vi "_OBSOLETE_PathPlanner_Trajectory_JoinSplines.vi"(9 "Step":dbl, 10 "Max Velocity":dbl, 11 "PathPoints":T5[](array[typedef]) {"HolonomicRotation"."SIN" format="%13.4f"; "HolonomicRotation"."COS" format="%13.4f"; "HolonomicRotation"."VALUE" format="%13.4f"; "NextControl"."Y" format="%14.3f"; "NextControl"."X" format="%14.3f"; "PrevControl"."Y" format="%14.3f"; "PrevControl"."X" format="%14.3f"; "AnchorPoint"."Y" format="%14.3f"; "AnchorPoint"."X" format="%14.3f"}) -> (3 "outPathPlannerStates":T1[](array[typedef]) {"TargetHolonomicRotation"."SIN" format="%13.4f"; "TargetHolonomicRotation"."COS" format="%13.4f"; "TargetHolonomicRotation"."VALUE" format="%13.4f"; "Heading"."SIN" format="%13.4f"; "Heading"."COS" format="%13.4f"; "Heading"."VALUE" format="%13.4f"; "PositionMeters"."Y" format="%14.3f"; "PositionMeters"."X" format="%14.3f"})   [LabVIEW 2019]
uses:
  <vilib>/Rock Robotics/WPI/ThirdParty/JAS_Junk/TrajLib/TypeDef/ROTATION2D.ctl
  <vilib>/Rock Robotics/WPI/ThirdParty/JAS_Junk/TrajLib/Trajectory_Library.lvlib
  <vilib>/Rock Robotics/WPI/ThirdParty/JAS_Junk/TrajLib/TypeDef/TRANSLATION2D.ctl
  TypeDef/PathPlannerTrajectoryState.ctl
  PathPlanner24.lvlib
  TypeDef/PathPlannerPathConstraints.ctl
  TypeDef/PathPlannerWaypoint.ctl
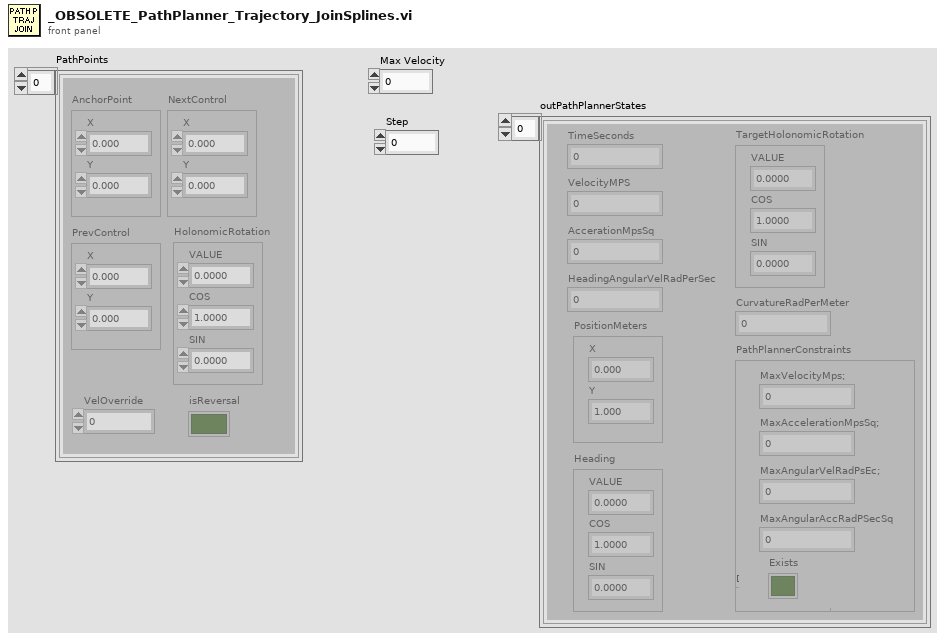
[diagram p1: front panel]
types:
  T1 = typedef "PathPlanner24.lvlib/PathPlannerTrajectoryState.ctl" = cluster{"TimeSeconds":dbl, "VelocityMPS":dbl, "AccerationMpsSq":dbl, "HeadingAngularVelRadPerSec":dbl, "PositionMeters":T2, "Heading":T3, "TargetHolonomicRotation":T3, "CurvatureRadPerMeter":dbl, "DeltaPos":dbl, "PathPlannerConstraints":T4}
  T2 = typedef "Trajectory_Library.lvlib/TRANSLATION2D.ctl" = cluster{"X":dbl, "Y":dbl}
  T3 = typedef "Trajectory_Library.lvlib/ROTATION2D.ctl" = cluster{"VALUE":dbl, "COS":dbl, "SIN":dbl}
  T4 = typedef "PathPlanner24.lvlib/PathPlannerPathConstraints.ctl" = cluster{"MaxVelocityMps;":dbl, "MaxAccelerationMpsSq;":dbl, "MaxAngularVelRadPsEc;":dbl, "MaxAngularAccRadPSecSq":dbl, "Exists":bool}
  T5 = typedef "PathPlanner24.lvlib/PathPlannerWaypoint.ctl" = cluster{"AnchorPoint":T2, "PrevControl":T2, "NextControl":T2, "HolonomicRotation":T3, "VelOverride":dbl, "isReversal":bool}
  T6 = typedef "Trajectory_Library.lvlib/POSE2D.ctl" = cluster{"TRANSLATION":T2, "ROTATION":T3}
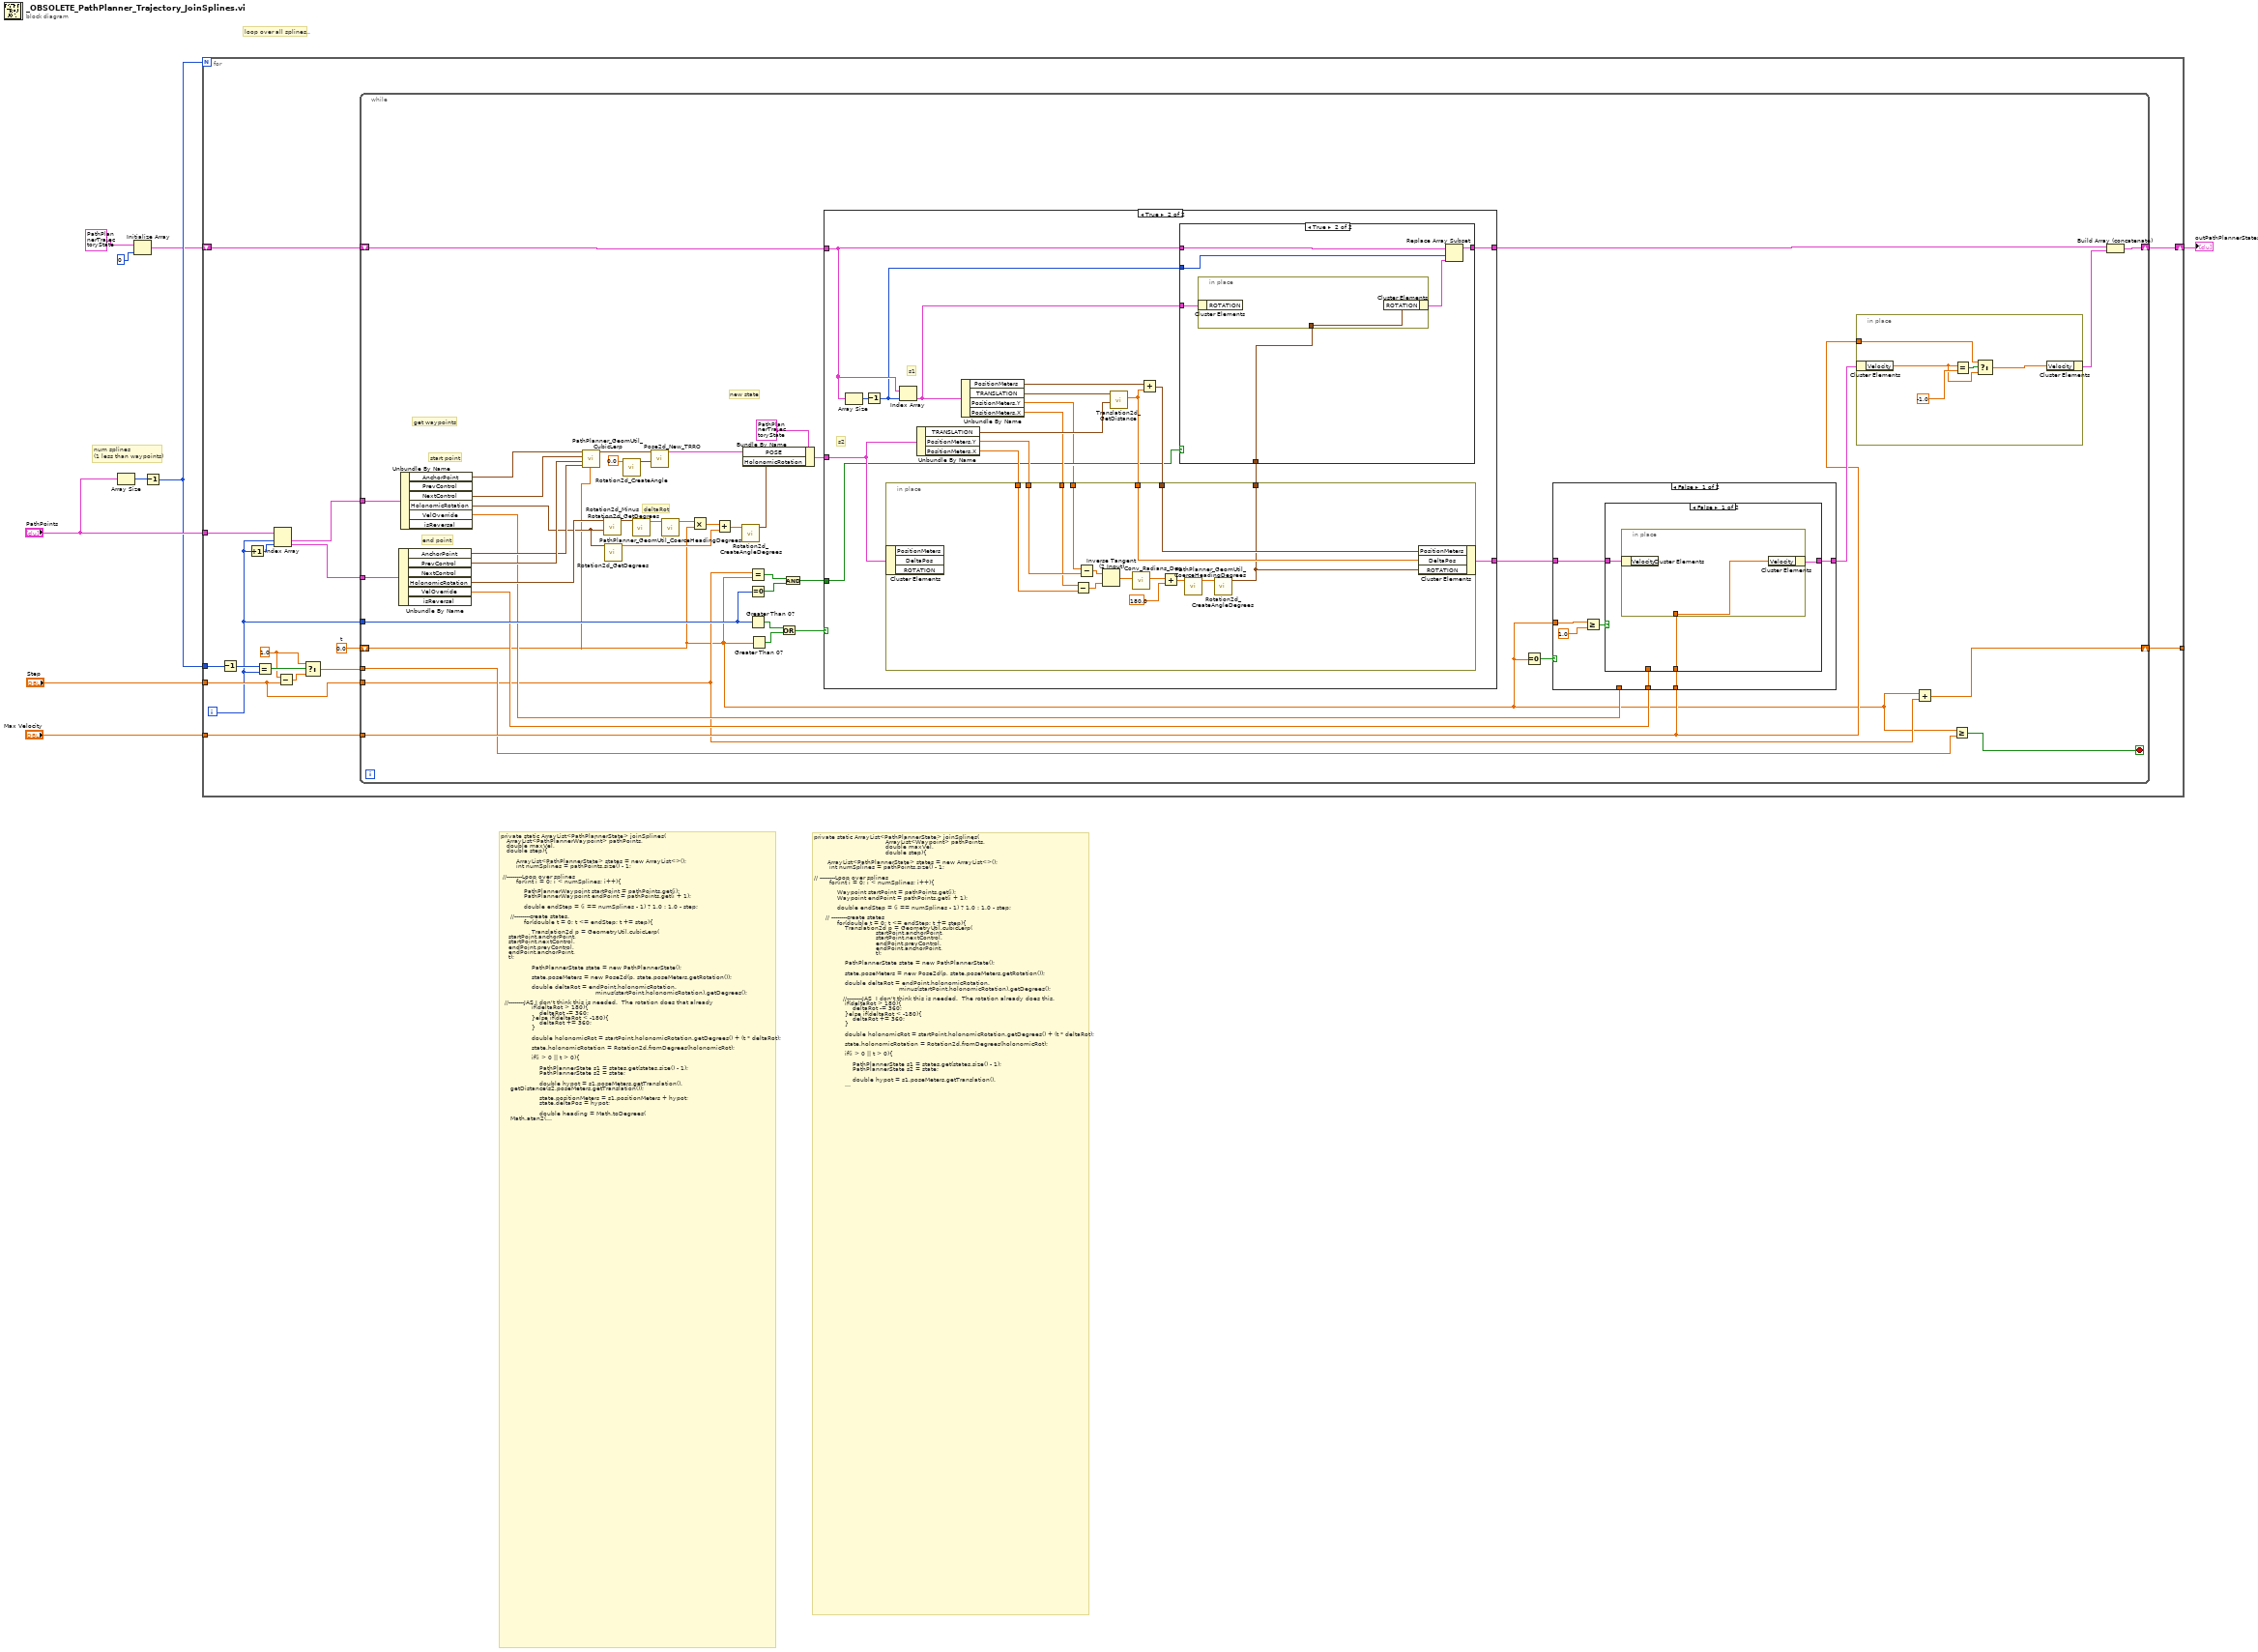
[diagram p0: block diagram]
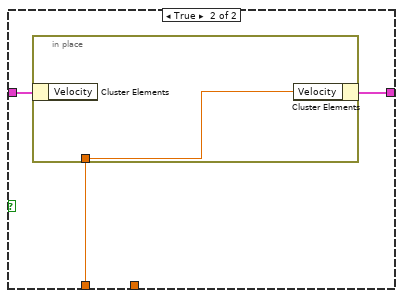
[diagram p2: hidden frame]
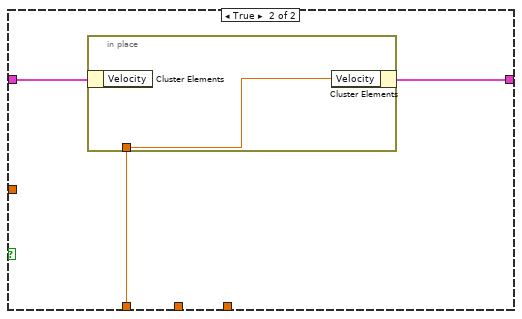
[diagram p3: hidden frame]
diagram:
  # "private static ArrayList<PathPlannerState> joinSplines(\n                                     ArrayList<Waypoint> pathPoints, \n                                     double maxVel, \n                                     double step){\n \n       ArrayList<PathPlannerState> states = new ArrayList<>();\n        int numSplines = pathPoints.size() - 1;\n\n// --------Loop over splines\n        for(int i = 0; i < numSplines; i++){\n\n            Waypoint startPoint = pathPoints.get(i);\n            Waypoint endPoint = pathPoints.get(i + 1);\n\n            double endStep = (i == numSplines - 1) ? 1.0 : 1.0 - step;\n\n      // --------create states\n            for(double t = 0; t <= endStep; t += step){\n                Translation2d p = GeometryUtil.cubicLerp(\n                                startPoint.anchorPoint, \n                                startPoint.nextControl, \n                                endPoint.prevControl, \n                                endPoint.anchorPoint, \n                                t);\n\n                PathPlannerState state = new PathPlannerState();\n\n                state.poseMeters = new Pose2d(p, state.poseMeters.getRotation());\n\n                double deltaRot = endPoint.holonomicRotation.\n                                            minus(startPoint.holonomicRotation).getDegrees();\n\n               //--------JAS  I don't think this is needed.  The rotation already does this.\n                if(deltaRot > 180){\n                    deltaRot -= 360;\n                }else if(deltaRot < -180){\n                    deltaRot += 360;\n                }\n\n                double holonomicRot = startPoint.holonomicRotation.getDegrees() + (t * deltaRot);\n\n                state.holonomicRotation = Rotation2d.fromDegrees(holonomicRot);\n\n                if(i > 0 || t > 0){\n\n                    PathPlannerState s1 = states.get(states.size() - 1);\n                    PathPlannerState s2 = state;\n\n                    double hypot = s1.poseMeters.getTranslation().\n                                                   getDistance(s2.poseMeters.getTranslation());\n\n                    state.positionMeters = s1.positionMeters + hypot;\n                    state.deltaPos = hypot;\n\n                    double heading = Math.toDegrees(\n                                                          Math.atan2(\n                                                                s1.poseMeters.getY() - s2.poseMeters.getY(), \n                                                               s1.poseMeters.getX() - s2.poseMeters.getX()\n                                                          )) + 180;\n\n                    if(heading > 180){\n                        heading -= 360;\n                    }else if(heading < -180){\n                        heading += 360;\n                    }\n\n                    state.poseMeters = new Pose2d(\n                                                        state.poseMeters.getTranslation(), \n                                                        Rotation2d.fromDegrees(heading));\n\n                    if(i == 0 && t == step){\n                        states.get(states.size() - 1).poseMeters = new Pose2d(\n                                                     states.get(states.size() - 1).poseMeters.getTranslation(), \n                                                     Rotation2d.fromDegrees(heading));\n                    }\n                }\n\n                if(t == 0.0){\n                    state.velocityMetersPerSecond = startPoint.velOverride;\n                }else if(t >= 1.0){\n                    state.velocityMetersPerSecond = endPoint.velOverride;\n                }else {\n                    state.velocityMetersPerSecond = maxVel;\n                }\n\n                if(state.velocityMetersPerSecond == -1) state.velocityMetersPerSecond = maxVel;\n\n                states.add(state);\n            }\n        }\n        return states;\n    }"
  # "private static ArrayList<PathPlannerState> joinSplines(\n\t\t\tArrayList<PathPlannerWaypoint> pathPoints, \n\t\t\tdouble maxVel, \n\t\t\tdouble step){\n\n        ArrayList<PathPlannerState> states = new ArrayList<>();\n        int numSplines = pathPoints.size() - 1;\n\n\t//--------Loop over splines\n        for(int i = 0; i < numSplines; i++){\n\n            PathPlannerWaypoint startPoint = pathPoints.get(i);\n            PathPlannerWaypoint endPoint = pathPoints.get(i + 1);\n\n            double endStep = (i == numSplines - 1) ? 1.0 : 1.0 - step;\n\n\t    //--------create states.\n            for(double t = 0; t <= endStep; t += step){\n\n                Translation2d p = GeometryUtil.cubicLerp(\n\t\t\t\tstartPoint.anchorPoint, \n\t\t\t\tstartPoint.nextControl, \n\t\t\t\tendPoint.prevControl, \n\t\t\t\tendPoint.anchorPoint, \n\t\t\t\tt);\n\n                PathPlannerState state = new PathPlannerState();\n\n                state.poseMeters = new Pose2d(p, state.poseMeters.getRotation());\n\n                double deltaRot = endPoint.holonomicRotation.\n\t                                            \t\t\t\tminus(startPoint.holonomicRotation).getDegrees();\n\n\t\t//--------JAS I don't think this is needed.  The rotation does that already\n                if(deltaRot > 180){\n                    deltaRot -= 360;\n                }else if(deltaRot < -180){\n                    deltaRot += 360;\n                }\n\n                double holonomicRot = startPoint.holonomicRotation.getDegrees() + (t * deltaRot);\n\n                state.holonomicRotation = Rotation2d.fromDegrees(holonomicRot);\n\n                if(i > 0 || t > 0){\n\n                    PathPlannerState s1 = states.get(states.size() - 1);\n                    PathPlannerState s2 = state;\n\n                    double hypot = s1.poseMeters.getTranslation().\n\t\t\t\t\tgetDistance(s2.poseMeters.getTranslation());\n\n                    state.positionMeters = s1.positionMeters + hypot;\n                    state.deltaPos = hypot;\n\n                    double heading = Math.toDegrees(\n\t\t\t\t\tMath.atan2(\n\t\t\t\t\t\ts1.poseMeters.getY() - s2.poseMeters.getY(),\n\t\t\t\t\t\t s1.poseMeters.getX() - s2.poseMeters.getX()\n\t\t\t\t\t))  + 180;\n\n                    if(heading > 180){\n                        heading -= 360;\n                    }else if(heading < -180){\n                        heading += 360;\n                    }\n\n                    state.poseMeters = new Pose2d(\n\t\t\t\t\tstate.poseMeters.getTranslation(), \n\t\t\t\t\tRotation2d.fromDegrees(heading));\n\n                    if(i == 0 && t == step){\n                        states.get(states.size() - 1).poseMeters = new Pose2d(\n\t\t\t\t\tstates.get(states.size() - 1).poseMeters.getTranslation(),\n\t\t\t\t\tRotation2d.fromDegrees(heading));\n                    }\n                }  \n\n                if(t == 0.0){\n                    state.velocityMetersPerSecond = startPoint.velOverride;\n                }else if(t >= 1.0){  //  V2022.01  }else if(t == 1.0){\n                    state.velocityMetersPerSecond = endPoint.velOverride;\n                }else {\n                    state.velocityMetersPerSecond = maxVel;\n                }\n\n                if(state.velocityMetersPerSecond == -1) \n\t\t\tstate.velocityMetersPerSecond = maxVel;\n\n                states.add(state);\n\n\n            }  // ---- end of state loop\n        }  // ---- end of spline loop\n        return states;\n    }"
  # "loop over all splines.."
  # "num splines\n(1 less than waypoints)"
  n1 = Array Size(array="PathPoints") -> (size(s)=w9:i32)
  n2 = Initialize Array(T1 {"TimeSeconds"=0.0, "VelocityMPS"=0.0, "AccerationMpsSq"=0.0, "HeadingAngularVelRadPerSec"=0.0, "PositionMeters"={"X"=0.0, "Y"=1.0}, "Heading"={"VALUE"=0.0, "COS"=1.0, "SIN"=0.0}, "TargetHolonomicRotation"={"VALUE"=0.0, "COS"=1.0, "SIN"=0.0}, "CurvatureRadPerMeter"=0.0, "DeltaPos"=0.0, "PathPlannerConstraints"={"MaxVelocityMps;"=0.0, "MaxAccelerationMpsSq;"=0.0, "MaxAngularVelRadPsEc;"=0.0, "MaxAngularAccRadPSecSq"=0.0, "Exists"=FALSE}} ("PathPlannerState"), 0 ("dimension size")) -> (w3:T1[])
  n3 = Decrement(x=w9) -> (x-1=w7:i32)
  n4 = for {
    N: w7 -> [_]
    tunnel: "PathPoints" -> [w20]
    tunnel: w7 -> [w25]
    tunnel: "Step" -> [w17]
    tunnel: "Max Velocity" -> [w13]
    shift-right: [w11] -> w2
    shift-left: w3 -> [w12]
    tunnel: [w10] -> _
    i -> [w14]
    w19 = 0.0  # t
    w21 = 1.0
    n5 = Decrement(x=w25) -> (x-1=w24:i32)
    n6 = Increment(x=w14) -> (x+1=w26:i32)
    n7 = Equal?(x=w24, y=w14) -> (x = y?=w23:bool)
    n8 = Index Array(array=w20, index #1=w14, index #2=w26) -> (element #1=w16:T5, element #2=w15:T5)
    n9 = Subtract(x=w21, y=w17) -> (x-y=w22:dbl)
    n10 = Select(t=w21, s=w23, f=w22) -> (s? t:f=w18:dbl)
    n11 = while {
      tunnel: w18 -> [w31]
      tunnel: w17 -> [w29]
      tunnel: w16 -> [w67]
      tunnel: w15 -> [w66]
      shift-right: [w68] -> w11
      shift-left: w12 -> [w46]
      tunnel: w14 -> [w42]
      tunnel: w13 -> [w33]
      shift-right: [w28] -> w10
      shift-left: w19 -> [w27]
      stop <- w30 stop-if-true
      # "get waypoints"
      # "new state"
      # "deltaRot"
      # "end point"
      # "start point"
      n12 = Unbundle By Name(w66) -> ("AnchorPoint"=w62:T2, "PrevControl"=w63:T2, "HolonomicRotation"=w61:T3, "VelOverride"=w35:dbl)  [unwired: 2 out]
      n13 = Unbundle By Name(w67) -> ("AnchorPoint"=w65:T2, "NextControl"=w64:T2, "HolonomicRotation"=w53:T3, "VelOverride"=w36:dbl)  [unwired: 2 out]
      n14 = call "PathPlanner_GeomUtil_CubicLerp.vi"("T"=w27, "D"=w62, "C"=w63, "B"=w64, "A"=w65) -> ("Lerp"=w55:T2)  [unwired: 6 in]
      n15 = call <vilib>:"Rotation2d_Minus.vi"("other ROTATION"=w53, "in ROTATION"=w61) -> ("out ROTATION"=w60:T3)  [unwired: 9 in]
      n16 = call <vilib>:"Rotation2d_GetDegrees.vi"("in ROTATION"=w53) -> ("AngleDegrees"=w51:dbl)  [unwired: 10 in]
      n17 = call <vilib>:"Rotation2d_CreateAngle.vi"("Angle"=0.0) -> ("ROTATION"=w57:T3)  [unwired: 10 in]
      n18 = call <vilib>:"Rotation2d_GetDegrees.vi"("in ROTATION"=w60) -> ("AngleDegrees"=w59:dbl)  [unwired: 10 in]
      n19 = call <vilib>:"Pose2d_New_TRRO.vi"("ROTATION"=w57, "TRANSLATION"=w55) -> ("outPOSE"=w54:T6)  [unwired: 9 in]
      n20 = call "PathPlanner_GeomUtil_CoerceHeadingDegrees.vi"("in Degrees"=w59) -> ("out Degrees"=w58:dbl)  [unwired: 10 in]
      n21 = Multiply(x=w58, y=w27) -> (x*y=w52:dbl)
      n22 = Add(x=w52, y=w51) -> (x+y=w50:dbl)
      n23 = call <vilib>:"Rotation2d_CreateAngleDegrees.vi"("Angle_Degrees"=w50) -> ("ROTATION"=w45:T3)  [unwired: 10 in]
      n24 = Bundle By Name(cluster=T1 {"TimeSeconds"=0.0, "VelocityMPS"=0.0, "AccerationMpsSq"=0.0, "HeadingAngularVelRadPerSec"=0.0, "PositionMeters"={"X"=0.0, "Y"=1.0}, "Heading"={"VALUE"=0.0, "COS"=1.0, "SIN"=0.0}, "TargetHolonomicRotation"={"VALUE"=0.0, "COS"=1.0, "SIN"=0.0}, "CurvatureRadPerMeter"=0.0, "DeltaPos"=0.0, "PathPlannerConstraints"={"MaxVelocityMps;"=0.0, "MaxAccelerationMpsSq;"=0.0, "MaxAngularVelRadPsEc;"=0.0, "MaxAngularAccRadPSecSq"=0.0, "Exists"=FALSE}} ("PathPlannerState"), "POSE"=w54, "HolonomicRotation"=w45) -> (w44:T1)
      n25 = Equal?(x=w29, y=w27) -> (x = y?=w41:bool)
      n26 = Equal To 0?(x=w42) -> (x = 0?=w40:bool)
      n27 = Greater Than 0?(x=w42) -> (x > 0?=w49:bool)
      n28 = Greater Than 0?(x=w27) -> (x > 0?=w48:bool)
      n29 = Or(x=w49, y=w48) -> (x .or. y?=w47:bool)
      n30 = And(x=w41, y=w40) -> (x .and. y?=w39:bool)
      n31 = case shown="True" w47 {
        tunnel: w46 -> [w94 w103]
        tunnel: w44 -> [w95 w111]
        tunnel: [w94 w102] -> w43
        tunnel: [w95 w104] -> w37
        tunnel: w39 -> [_ w101]
        frame False {
        }
        frame True {
          # "s2"
          # "s1"
          n32 = Array Size(array=w103) -> (size(s)=w113:i32)
          n33 = Decrement(x=w113) -> (x-1=w100:i32)
          n34 = Index Array(array=w103, index=w100) -> (element=w98:T1)
          n35 = Unbundle By Name(w111) -> ("TRANSLATION"=w112:T2, "PositionMeters.Y"=w107:dbl, "PositionMeters.X"=w105:dbl)
          n36 = Unbundle By Name(w98) -> ("PositionMeters"=w110:T2, "TRANSLATION"=w99:T2, "PositionMeters.Y"=w96:dbl, "PositionMeters.X"=w106:dbl)
          n37 = call <vilib>:"Translation2d_GetDistance.vi"("other Translation"=w112, "In Translation"=w99) -> ("Distance"=w108:dbl)  [unwired: 9 in]
          n38 = Add(x=w110, y=w108) -> (x+y=w109:T2)
          n39 = in-place {
            in-place-border: w109 -> [w135]
            in-place-border: w108 -> [w134]
            in-place-border: w96 -> [w133]
            in-place-border: w107 -> [w132]
            in-place-border: w106 -> [w131]
            in-place-border: w105 -> [w130]
            in-place-border: [w122] -> w97
            n40 = in-place-cluster #1(w111) -> ()  [unwired: 3 out]
            n41 = Subtract(x=w131, y=w130) -> (x-y=w128:dbl)
            n42 = Subtract(x=w133, y=w132) -> (x-y=w129:dbl)
            n43 = Inverse Tangent (2 Input)(1:w128, 2:w129) -> (0:w127:dbl)
            n44 = call <vilib>:"Conv_Radians_Deg.vi"("Radians"=w127) -> ("Degrees"=w126:dbl)  [unwired: 10 in]
            n45 = Add(x=w126, y=180.0) -> (x+y=w124:dbl)
            n46 = call "PathPlanner_GeomUtil_CoerceHeadingDegrees.vi"("in Degrees"=w124) -> ("out Degrees"=w123:dbl)  [unwired: 10 in]
            n47 = call <vilib>:"Rotation2d_CreateAngleDegrees.vi"("Angle_Degrees"=w123) -> ("ROTATION"=w122:T3)  [unwired: 10 in]
            n48 = in-place-cluster #1("PositionMeters"=w135, "DeltaPos"=w134, "ROTATION"=w122) -> (w104:T1)
          }
          n49 = case shown="True" w101 {
            tunnel: w103 -> [w114 w120]
            tunnel: [w114 w116] -> w102
            tunnel: w100 -> [_ w118]
            tunnel: w98 -> [_ w119]
            tunnel: w97 -> [_ w115]
            frame False {
            }
            frame True {
              n50 = in-place {
                in-place-border: w115 -> [w121]
                n51 = in-place-cluster #2(w119) -> ()  [unwired: 1 out]
                n52 = in-place-cluster #2("ROTATION"=w121) -> (w117:T1)
              }
              n53 = Replace Array Subset(array=w120, new element=w117, index=w118) -> (w116:T1[])
            }
          }
        }
      }
      n54 = Equal To 0?(x=w27) -> (x = 0?=w38:bool)
      n55 = case shown="False" w38 {
        tunnel: w27 -> [w75 _]
        tunnel: w37 -> [w80 w92]
        tunnel: w36 -> [_ w91]
        tunnel: w35 -> [w79 _]
        tunnel: [w78 w90] -> w34
        tunnel: w33 -> [w77 _]
        frame False {
          n56 = Greater Or Equal?(x=w75, y=1.0) -> (x >= y?=w81:bool)
          n57 = case shown="False" w81 {
            tunnel: w80 -> [w84 w88]
            tunnel: w79 -> [_ w87]
            tunnel: [w83 w86] -> w78
            tunnel: w77 -> [w82 _]
            frame False {
              n58 = in-place {
                in-place-border: w82 -> [w85]
                n59 = in-place-cluster #3(w84) -> ()  [unwired: 1 out]
                n60 = in-place-cluster #3("Velocity"=w85) -> (w83:T1)
              }
            }
            frame True {
              n61 = in-place {
                in-place-border: w87 -> [w89]
                n62 = in-place-cluster #4(w88) -> ()  [unwired: 1 out]
                n63 = in-place-cluster #4("Velocity"=w89) -> (w86:T1)
              }
            }
          }
        }
        frame True {
          n64 = in-place {
            in-place-border: w91 -> [w93]
            n65 = in-place-cluster #5(w92) -> ()  [unwired: 1 out]
            n66 = in-place-cluster #5("Velocity"=w93) -> (w90:T1)
          }
        }
      }
      n67 = in-place {
        in-place-border: w33 -> [w70]
        n68 = in-place-cluster #6(w34) -> ("Velocity"=w72:dbl)
        n69 = Equal?(x=w72, y=-1.0) -> (x = y?=w73:bool)
        n70 = Select(t=w70, s=w73, f=w72) -> (s? t:f=w71:dbl)
        n71 = in-place-cluster #6("Velocity"=w71) -> (w32:T1)
      }
      n72 = Add(x=w27, y=w29) -> (x+y=w28:dbl)
      n73 = Greater Or Equal?(x=w27, y=w31) -> (x >= y?=w30:bool)
      n74 = Build Array (concatenate)(w43, w32) -> (w68:T1[])
    }
  }
  "outPathPlannerStates" <- w2
